vi "Example_application.vi"() -> ()   [LabVIEW 2016, in "OSB_uMp_library.lvlib"]
doc: "Example VI to show how to use this LabVIEW library for control of a Sensapex uMp manipulator."
uses:
  OSB_uMp_library.lvlib
panel:
  out "uMp version":i32[](array[numeric])
  out "error out":errorcluster
  in  "Quit":bool
  in  "x,y,z step (nm)":i32[](array[numeric])=[1000000, 1000000, 1000000]
  in  "Go to position (nm)":i32[](array[numeric])=[10000000, 10000000, 10000000]
  in  "Step":bool
  in  "Go to":bool
  in  "Stop uMp":bool
  in  "Go to home":bool
  in  "Set home":bool
  in  "Calibrate":bool caption="Device will move over full range of motion!"
  out "XYZ position (nm)":cluster{"x_pos":i32, "y_pos":i32, "z_pos":i32}
  out "uMp moving?":bool
  in  "Speed (um/s)":i32=500
  in  "Device ID":i32=1
  in  "Connect":bool
  in  "uMp UDP address":string="169.254.255.255"
  # "SETUP"
  # "STATUS"
  # "UMP CONTROL"
  # "By Stuart Box at OxSyBio Ltd, 2017\n\nThis software is provided WITHOUT ANY WARRANTY; without even the implied warranty of MERCHANTABILITY or FITNESS FOR A PARTICULAR PURPOSE.\n\ninfo@oxsybio.com\n\nOxSyBio Ltd, The Walbrook Building, 25 Walbrook, London, EC4N 8AF"
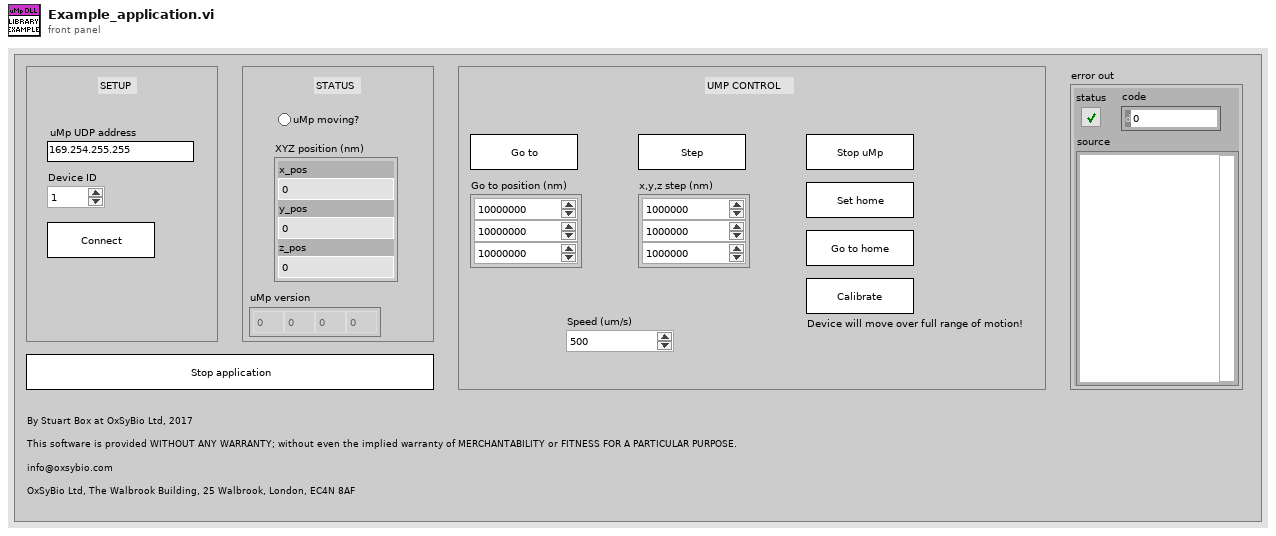
[diagram p1: front panel]
types:
  T1 = enum8{"Enabled", "Disabled", "Disabled and Grayed Out"}
  T2 = cluster{"Handle":i64, "Device ID":i32, "Speed (um/s)":i32, "Connected?":bool}
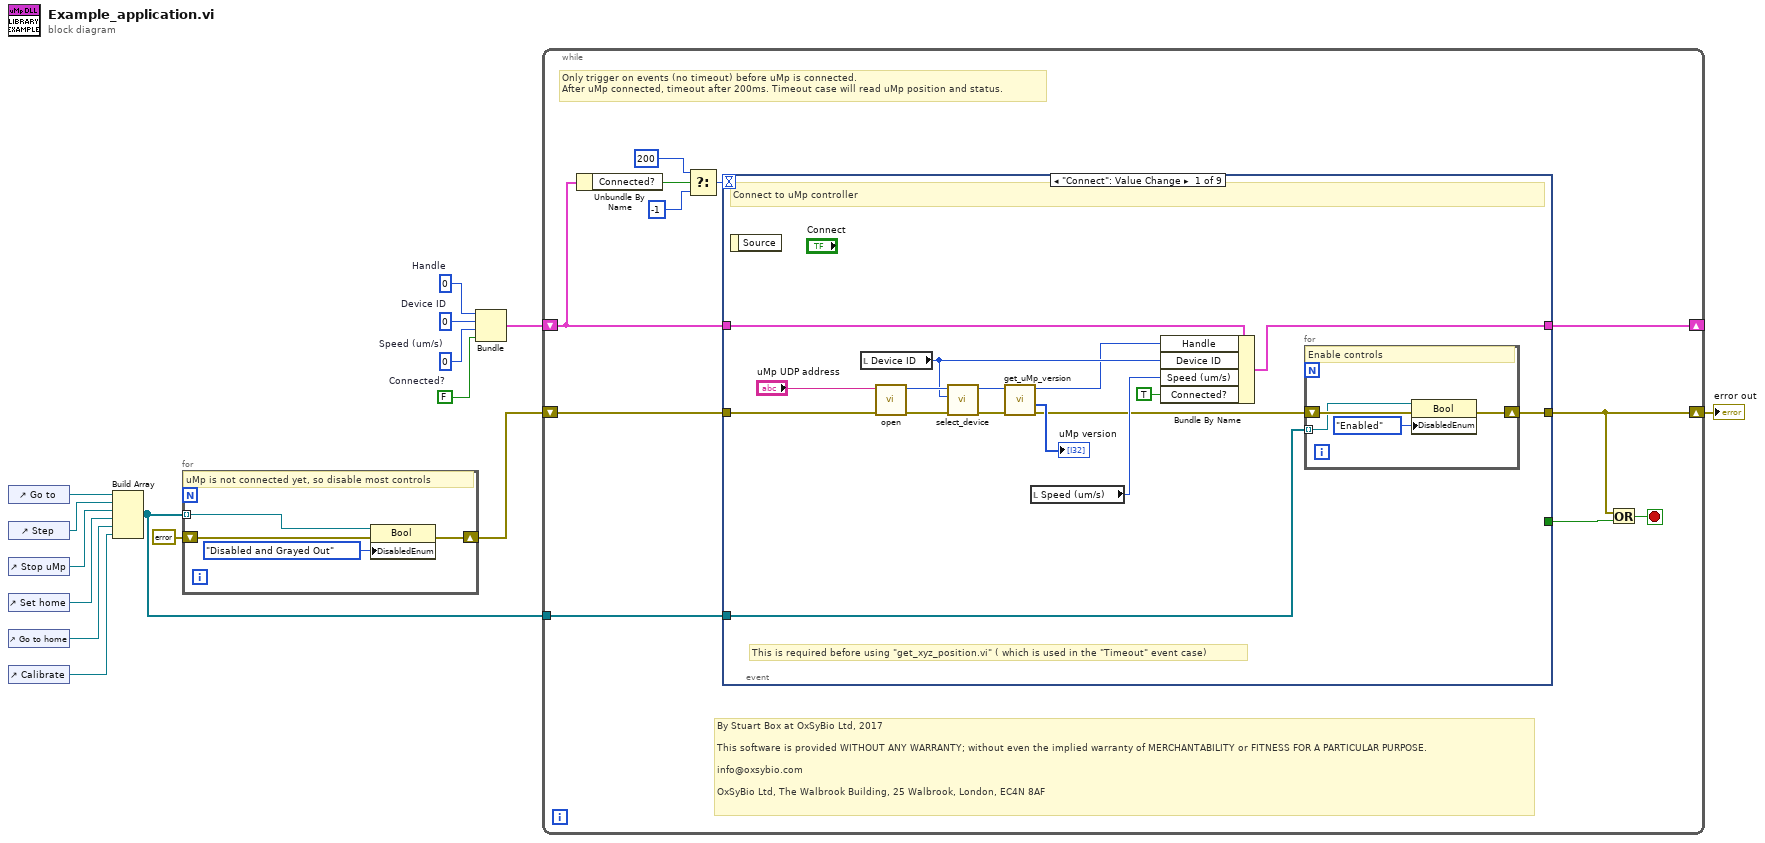
[diagram p0: block diagram]
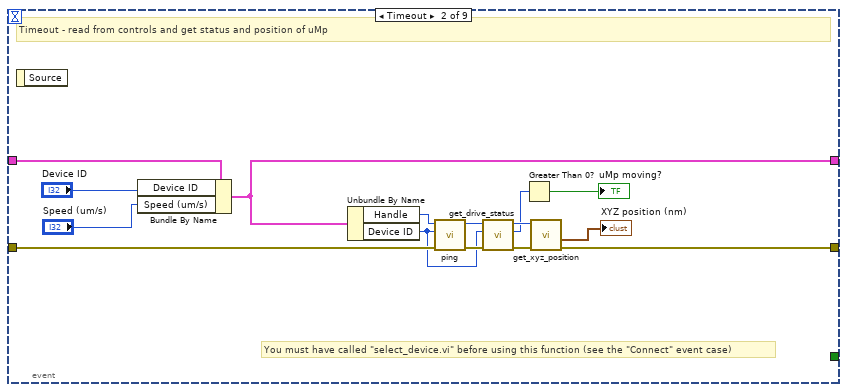
[diagram p2: hidden frame]
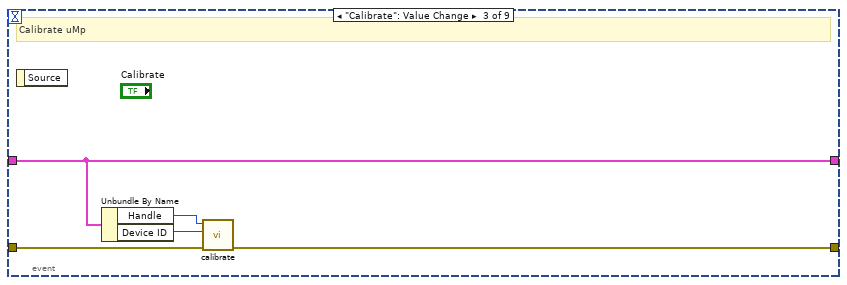
[diagram p3: hidden frame]
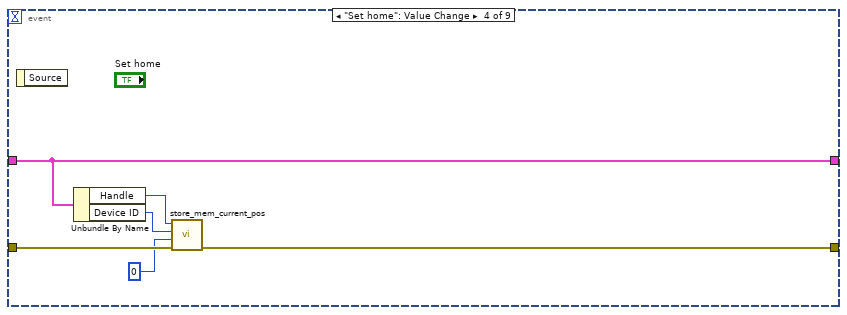
[diagram p4: hidden frame]
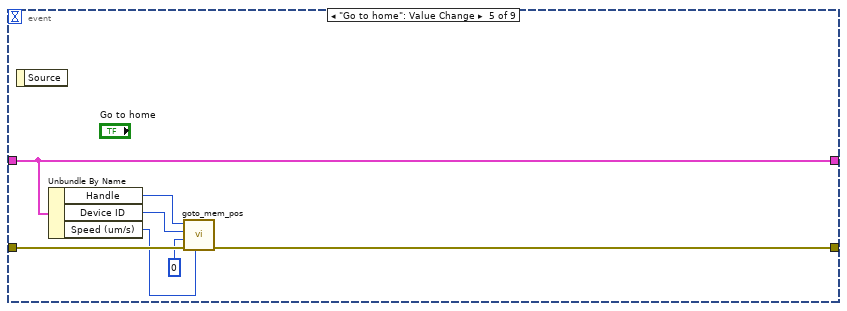
[diagram p5: hidden frame]
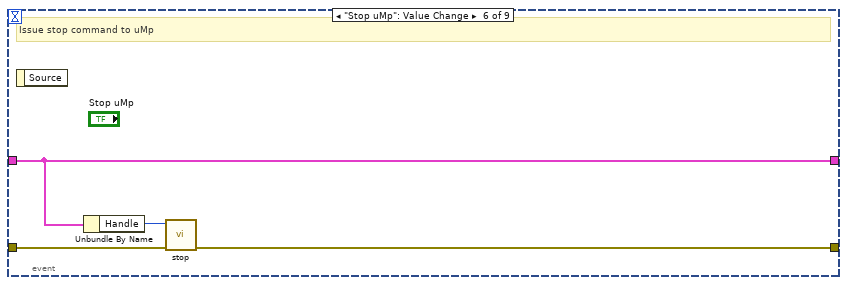
[diagram p6: hidden frame]
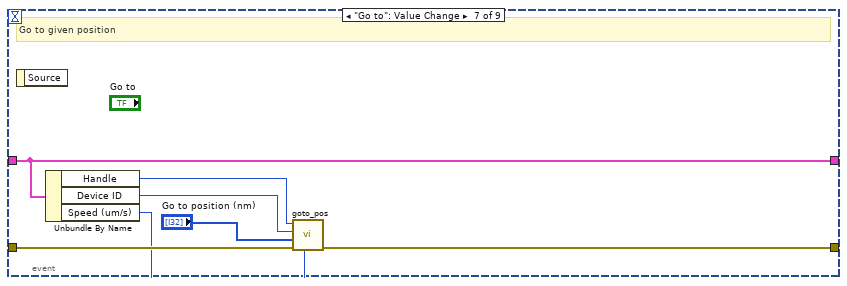
[diagram p7: hidden frame]
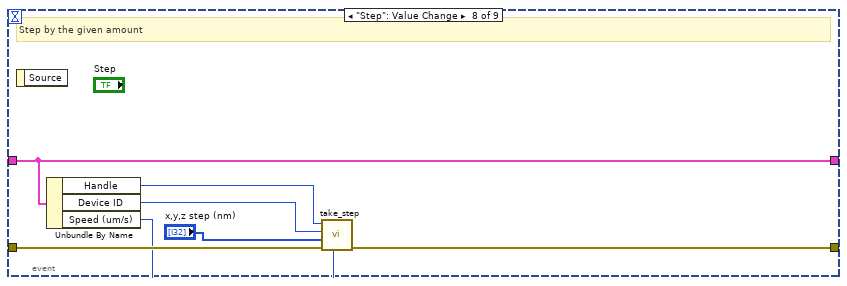
[diagram p8: hidden frame]
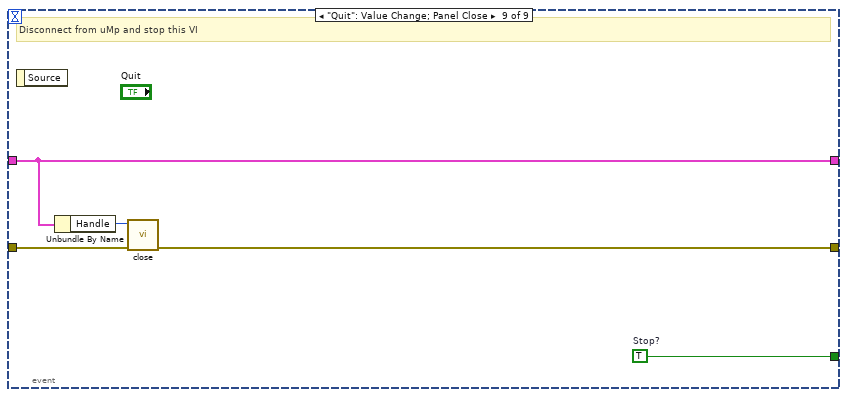
[diagram p9: hidden frame]
diagram:
  w10 = FALSE  # Connected?
  w13 = 0  # Speed (um/s)
  w14 = 0  # Device ID
  w15 = i64 0  # Handle
  n1 = control-ref of="Go to"() -> (w9:refnum<vi>)
  n2 = control-ref of="Step"() -> (w4:refnum<vi>)
  n3 = control-ref of="Stop uMp"() -> (w5:refnum<vi>)
  n4 = control-ref of="Set home"() -> (w6:refnum<vi>)
  n5 = control-ref of="Go to home"() -> (w7:refnum<vi>)
  n6 = control-ref of="Calibrate"() -> (w8:refnum<vi>)
  n7 = Build Array(w9, w4, w5, w6, w7, w8) -> (w1:refnum<vi>[])
  n8 = for {
    tunnel: w1 -> [w19] mode=indexing
    shift-right: [w17] -> w3
    shift-left: errorcluster {"status"=FALSE, "code"=0, "source"=""} ("error out") -> [w16]
    # "uMp is not connected yet, so disable most controls"
    n9 = property class="Bool"(reference=w19, error in=w16, "DisabledEnum"=T1."Disabled and Grayed Out" ("Disabled")) -> (error out=w17:errorcluster)  [unwired: 1 out]
  }
  n10 = Bundle("Handle"=w15, "Device ID"=w14, "Speed (um/s)"=w13, "Connected?"=w10) -> (w12:T2)  [unwired: 1 in]
  n11 = while {
    shift-right: [w27] -> w11
    shift-left: w3 -> [w30]
    shift-right: [w29] -> _
    shift-left: w12 -> [w25]
    tunnel: w1 -> [w20]
    stop <- w26 stop-if-true
    # "Only trigger on events (no timeout) before uMp is connected.\nAfter uMp connected, timeout after 200ms. Timeout case will read uMp position and status."
    # "By Stuart Box at OxSyBio Ltd, 2017\n\nThis software is provided WITHOUT ANY WARRANTY; without even the implied warranty of MERCHANTABILITY or FITNESS FOR A PARTICULAR PURPOSE.\n\ninfo@oxsybio.com\n\nOxSyBio Ltd, The Walbrook Building, 25 Walbrook, London, EC4N 8AF"
    n12 = Unbundle By Name(w25) -> ("Connected?"=w23:bool)
    n13 = Select(t=200, s=w23, f=-1) -> (s? t:f=w24:i32)
    n14 = event shown="[0] \"Connect\": Value Change" {
      selector: _ -> [_ _ _ _ _ _ _ _ _]
      dyn-events: _ -> [_ _ _ _ _ _ _ _ _]
      timeout: w24 -> [_ _ _ _ _ _ _ _ _]
      tunnel: w30 -> [w46 w62 w70 w76 w81 w87 w94 w101 w106]
      tunnel: [w32 w59 w69 w72 w80 w86 w89 w100 w104] -> w27
      tunnel: w25 -> [w44 w65 w66 w71 w83 w84 w88 w99 w103]
      tunnel: [w43 w58 w66 w71 w83 w84 w88 w99 w103] -> w29
      tunnel: [_ _ _ _ _ _ _ _ w102] -> w28
      tunnel: w20 -> [w31 _ _ _ _ _ _ _ _]
      event "Connect": Value Change {
        # "This is required before using \"get_xyz_position.vi\" ( which is used in the \"Timeout\" event case)"
        # "Connect to uMp controller"
        n15 = event-data() -> ()  [unwired: 1 in, 1 out]
        n16 = local read "Device ID"() -> (w39:i32)
        n17 = call "open.vi"("error in (no error)"=w46, "UDP target address (169.254.255.255)"="uMp UDP address") -> ("error out"=w41:errorcluster, "Handle out"=w40:i64)  [unwired: 8 in]
        n18 = call "select_device.vi"("error in (no error)"=w41, "device (1)"=w39, "Handle in"=w40) -> ("error out"=w38:errorcluster, "Handle out"=w37:i64)  [unwired: 6 in, 1 out]
        n19 = call "get_uMp_version.vi"("error in (no error)"=w38, "Handle in"=w37) -> ("error out"=w33:errorcluster, "uMp version"=→"uMp version":i32[], "Handle out"=w34:i64)  [unwired: 6 in, 1 out]
        n20 = local read "Speed (um/s)"() -> (w42:i32)
        n21 = Bundle By Name(cluster=w44, "Handle"=w34, "Device ID"=w39, "Speed (um/s)"=w42, "Connected?"=TRUE) -> (w43:T2)
        n22 = for {
          shift-right: [w49] -> w32
          shift-left: w33 -> [w48]
          tunnel: w31 -> [w47] mode=indexing
          # "Enable controls"
          n23 = property class="Bool"(reference=w47, error in=w48, "DisabledEnum"=T1."Enabled" ("Disabled")) -> (error out=w49:errorcluster)  [unwired: 1 out]
        }
      }
      event Timeout {
        # "You must have called \"select_device.vi\" before using this function (see the \"Connect\" event case)"
        # "Timeout - read from controls and get status and position of uMp"
        n24 = event-data() -> ()  [unwired: 1 in, 1 out]
        n25 = Bundle By Name(cluster=w65, "Device ID"="Device ID", "Speed (um/s)"="Speed (um/s)") -> (w58:T2)
        n26 = Unbundle By Name(w58) -> ("Handle"=w55:i64, "Device ID"=w54:i32)
        n27 = call "ping.vi"("error in (no error)"=w62, "Device ID"=w54, "Handle in"=w55) -> ("error out"=w61:errorcluster, "Handle out"=w57:i64)  [unwired: 6 in, 1 out]
        n28 = call "get_drive_status.vi"("error in (no error)"=w61, "Device ID"=w54, "Handle in"=w57) -> ("error out"=w60:errorcluster, "Return (<0 is error)"=w53:i32, "Handle out"=w56:i64)  [unwired: 6 in]
        n29 = Greater Than 0?(x=w53) -> (x > 0?=→"uMp moving?":bool)
        n30 = call "get_xyz_position.vi"("error in (no error)"=w60, "Handle in"=w56) -> ("error out"=w59:errorcluster, "XYZ position (nm)"=→"XYZ position (nm)":cluster{"x_pos":i32, "y_pos":i32, "z_pos":i32})  [unwired: 6 in, 2 out]
      }
      event "Calibrate": Value Change {
        # "Calibrate uMp"
        n31 = event-data() -> ()  [unwired: 1 in, 1 out]
        n32 = Unbundle By Name(w66) -> ("Handle"=w68:i64, "Device ID"=w67:i32)
        n33 = call "calibrate.vi"("error in (no error)"=w70, "device (1)"=w67, "Handle in"=w68) -> ("error out"=w69:errorcluster)  [unwired: 6 in, 2 out]
      }
      event "Set home": Value Change {
        n34 = event-data() -> ()  [unwired: 1 in, 1 out]
        n35 = Unbundle By Name(w71) -> ("Handle"=w75:i64, "Device ID"=w74:i32)
        n36 = call "store_mem_current_pos.vi"("error in (no error)"=w76, "storage_id"=0, "device ID"=w74, "Handle in"=w75) -> ("error out"=w72:errorcluster)  [unwired: 5 in, 2 out]
      }
      event "Go to home": Value Change {
        n37 = event-data() -> ()  [unwired: 1 in, 1 out]
        n38 = Unbundle By Name(w83) -> ("Handle"=w82:i64, "Device ID"=w79:i32, "Speed (um/s)"=w77:i32)
        n39 = call "goto_mem_pos.vi"("Speed (um/s)"=w77, "error in (no error)"=w81, "storage_id"=0, "device ID"=w79, "Handle in"=w82) -> ("error out"=w80:errorcluster)  [unwired: 4 in, 2 out]
      }
      event "Stop uMp": Value Change {
        # "Issue stop command to uMp"
        n40 = event-data() -> ()  [unwired: 1 in, 1 out]
        n41 = Unbundle By Name(w84) -> ("Handle"=w85:i64)
        n42 = call "stop.vi"("error in (no error)"=w87, "Handle in"=w85) -> ("error out"=w86:errorcluster)  [unwired: 7 in, 2 out]
      }
      event "Go to": Value Change {
        # "Go to given position"
        n43 = event-data() -> ()  [unwired: 1 in, 1 out]
        n44 = Unbundle By Name(w88) -> ("Handle"=w92:i64, "Device ID"=w91:i32, "Speed (um/s)"=w93:i32)
        n45 = call "goto_pos.vi"("Speed (um/s)"=w93, "error in (no error)"=w94, "New position (nm)"="Go to position (nm)", "device ID"=w91, "Handle in"=w92) -> ("error out"=w89:errorcluster)  [unwired: 4 in, 2 out]
      }
      event "Step": Value Change {
        # "Step by the given amount"
        n46 = event-data() -> ()  [unwired: 1 in, 1 out]
        n47 = Unbundle By Name(w99) -> ("Handle"=w98:i64, "Device ID"=w97:i32, "Speed (um/s)"=w96:i32)
        n48 = call "take_step.vi"("Speed (um/s)"=w96, "error in (no error)"=w101, "x,y,z step size (nm)"="x,y,z step (nm)", "device ID"=w97, "Handle in"=w98) -> ("error out"=w100:errorcluster)  [unwired: 4 in, 2 out]
      }
      event "Quit": Value Change; Panel Close {
        w102 = TRUE  # Stop?
        # "Disconnect from uMp and stop this VI"
        n49 = event-data() -> ()  [unwired: 1 in, 1 out]
        n50 = Unbundle By Name(w103) -> ("Handle"=w105:i64)
        n51 = call "close.vi"("error in (no error)"=w106, "Handle in"=w105) -> ("error out"=w104:errorcluster)  [unwired: 9 in]
      }
    }
    n52 = Or(x=w27, y=w28) -> (x .or. y?=w26:bool)
  }
  "error out" <- w11
